vi "WT500 IEC 2015 Setup.vi"(0 "VISA Input":refnum<visa-resource-name>, 1 "Wiring (0: 1P2W, 1P2W, 1P2W)":T1=1 items=["1P2W, 1P2W, 1P2W", "1P3W, 1P2W", "3P3W, 1P2W", "1P2W, 1P3W", "1P2W, 3P3W", "3P4W", "3V3A"], 5 "V Range (8: 1000V)":u16(ring)=6 items=["AUTO", "15", "30", "60", "100", "150", "300", "600", "1000", "7.5", "15", "30", "50", "75", "150", "300", "500"], 7 "I Range (7: 40A)":u16(ring)=7 items=["AUTO", "500 mA", "1 A", "2 A", "5 A", "10 A", "20 A", "40 A", "S-AUTO", "50 mV", "100 mV", "200 mV", "500 mV", "1 V", "2 V", "5 V", "10 V", "250 mA", "500 mA", "1 A", "2.5 A", "5 A", "10 A", "20 A", "25 mV", "50 mV", "100 mV", "250 mV", "500 mV", "1 V", "2.5 V", "5 V"], 9 "Update Rate (3: 500ms)":u16(ring)=2 items=["-", "100ms", "200ms", "500ms", "1s", "2s", "5s"], 11 "Error In":errorcluster, 12 "Start/Stop (False: Stop)":bool=TRUE) -> (4 "VISA resource name out":refnum<visa-resource-name>, 6 "Standby Power Header":string[][](array[string]), 8 "WT500 Label Array":string[](array[string]), 10 "Uthd:Element 1":dbl, 15 "Error Out":errorcluster)   [LabVIEW 2019]
uses:
  Type Definitions/WT500 Wiring Control.ctl
  <vilib>/Utility/error.llb/whitespace.ctl
  <vilib>/Instr/_visa.llb/VISA Open Access Mode.ctl
  LLBs/ykwt500.llb/YKWT500 Read Numeric (Normal).vi
panel:
  in  "Pole":u16(ring)=1 items=["NONE", "Element 1", "Element 2", "Element 3", "Sigma"]
  in  "Measurement":u16(ring)=1 items=["None", "Urms", "Umn", "Udc", "Urmn", "Uac", "Irms", "Imn", "Idc", "Irmn", "Iac", "P", "S", "Q", "Lambda", "Phi", "Freq U", "Freq I", "U +peak", "U -peak", "I +peak", "I -peak", "Cf U", "Cf I", "Time", "Wp", "Wp+", "Wp-", "q", "q+", "q-", "WS", "WQ", "Eta 1", "Eta 2", "F1", "F2", "F3", "F4", "F5", "F6", "F7", "F8", "U(k)", "I(k)", "P(k)", "S(k)", "Q(k)", "Lambda(k)", "Phi(k)", "Phi U(k)", "Phi I(k)", "Uhdf(k)", "Ihdf(k)", "Phdf(k)", "Uthd", "Ithd", "Pthd", "Phi Ui-Uj", "Phi Ui-Uk", "Phi Ui-Ii", "Phi Ui-Ij", "Phi Ui-Ik", "Delta 1", "Delta 2", "Delta 3", "Delta 4"]
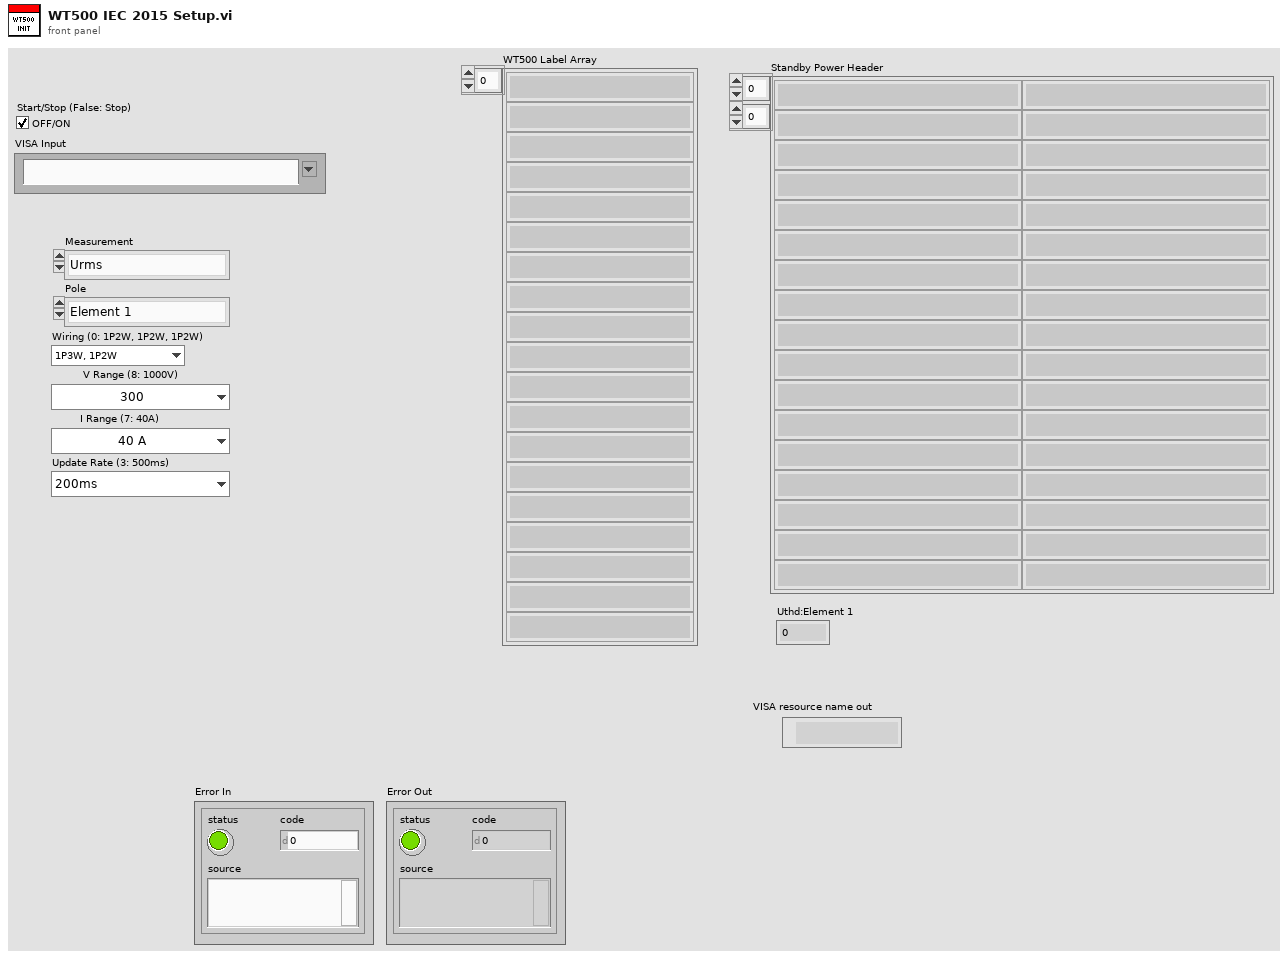
[diagram p1: front panel]
types:
  T1 = typedef "WT500 Wiring Control.ctl" = u16
  T2 = typedef "VISA Open Access Mode.ctl" = u32
  T3 = typedef "whitespace.ctl" = u16
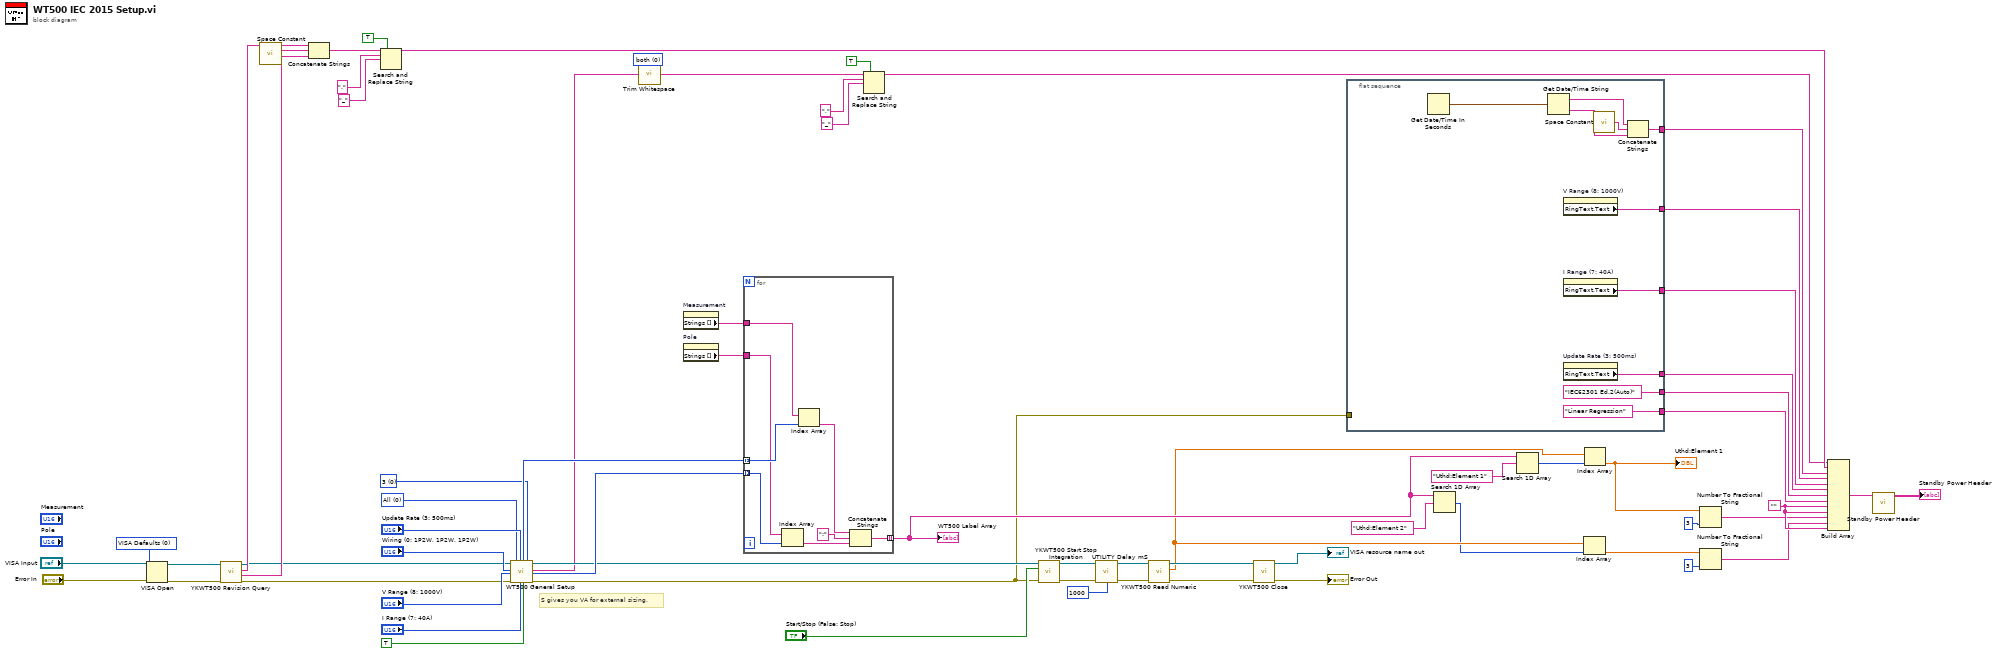
[diagram p0: block diagram]
diagram:
  w17 = T2 0 items=["VISA Defaults"=0, "Exclusive Lock"=1, "Load Configured Settings"=4] ("Access Mode")
  w18 = u16 0 items=["3", "6"] ("Crest Factor (0: 3)")
  w19 = u16 0 items=["All", "Element 1", "Element 2", "Element 3", "Sigma"] ("Element (0: All)")
  w25 = T3 0 items=["both", "start of string", "end of string"] ("location (both)")
  w45 = ""
  # "S gives you VA for external sizing."
  n1 = VISA Open(access mode=w17, error in (no error)="Error In", VISA resource name="VISA Input") -> (VISA resource name=w16:refnum<visa-resource-name>, error out=w15:errorcluster)  [unwired: 2 in]
  n2 = call "YKWT500 Revision Query.vi"("error in (no error)"=w15, "VISA resource name"=w16) -> ("error out"=w21:errorcluster, "Instrument Firmware Revision"=w52:string, "Instrument Driver Revision"=w53:string, "VISA resource name out"=w22:refnum<visa-resource-name>)  [unwired: 6 in]
  n3 = call <vilib>:"Space Constant.vi"() -> ("String"=w54:string)
  n4 = Concatenate Strings(w53, w54, w52) -> (w7:string)
  n5 = Search and Replace String(replace all?=TRUE ("replace all? (F)"), input string=w7, search string=",", replace string="_" ("replace string (\"\")")) -> (result string=w6:string)  [unwired: 4 in, 3 out]
  n6 = call "WT500 General Setup.vi"("VISA Refnum in"=w22, "Wiring (0: 1P2W, 1P2W, 1P2W)"="Wiring (0: 1P2W, 1P2W, 1P2W)", "V Range (8: 1000V)"="V Range (8: 1000V)", "error in (no error)"=w21, "Element (0: All)"=w19, "Update Rate (3: 500ms)"="Update Rate (3: 500ms)", "I Range (7: 40A)"="I Range (7: 40A)", "Reset Wh"=TRUE, "Crest Factor (0: 3)"=w18) -> ("Array of Measurements"=w63:u16[], "VISA Refnum out"=w58:refnum<visa-resource-name>, "Instrument ID"=w23:string, "Array Locations"=w64:u16[], "error out"=w26:errorcluster)  [unwired: 6 in]
  n7 = call <vilib>:"Trim Whitespace.vi"("string"=w23, "location (both)"=w25) -> ("trimmed string"=w2:string)
  n8 = property on="Measurement" class="Ring (strict)"() -> ("Strings []"=w60:string[])  [unwired: 2 in, 2 out]
  n9 = property on="Pole" class="Ring (strict)"() -> ("Strings []"=w59:string[])  [unwired: 2 in, 2 out]
  n10 = for {
    tunnel: w63 -> [w72] mode=indexing
    tunnel: w60 -> [w71]
    tunnel: w64 -> [w70] mode=indexing
    tunnel: w59 -> [w69]
    tunnel: [w65] -> w37 mode=indexing
    n11 = Index Array(array=w69, index=w70) -> (element=w66:string)
    n12 = Index Array(array=w71, index=w72) -> (element=w68:string)
    n13 = Concatenate Strings(w68, ":" ("string"), w66) -> (w65:string)
  }
  "WT500 Label Array" <- w37
  n14 = Search and Replace String(replace all?=TRUE ("replace all? (F)"), input string=w2, search string=",", replace string="_" ("replace string (\"\")")) -> (result string=w1:string)  [unwired: 4 in, 3 out]
  n15 = call "YKWT500 Start Stop Integration.vi"("error in (no error)"=w26, "Start/Stop (False: Stop)"="Start/Stop (False: Stop)", "VISA resource name"=w58) -> ("error out"=w29:errorcluster, "VISA resource name out"=w44:refnum<visa-resource-name>)  [unwired: 7 in]
  n16 = call "UTILITY Delay mS.vi"("Error In"=w29, "milliseconds to wait"=u32 1000) -> ("Error Out"=w28:errorcluster)  [unwired: 13 in]
  n17 = call-poly "YKWT500 Read Numeric.vi"("error in (no error)"=w28, "VISA resource name"=w44) -> ("error out"=w43:errorcluster, "Measurement Value"=w36:dbl[], "VISA resource name out"=w42:refnum<visa-resource-name>)  [unwired: 7 in]
  "VISA resource name out" <- w42
  n18 = call "YKWT500 Close.vi"("error in (no error)"=w43, "VISA resource name"=w42) -> ("error out"=→"Error Out":errorcluster)  [unwired: 9 in]
  n19 = flat-sequence {
    tunnel: [w78] -> w51
    tunnel: [w75] -> w50
    tunnel: [w74] -> w49
    tunnel: [w73] -> w48
    tunnel: ["IEC62301 Ed.2(Auto)" ("element")] -> w47
    tunnel: ["Linear Regression" ("element")] -> w46
    tunnel: w26 -> [_]
    frame #0 {
      n20 = Get Date/Time In Seconds() -> (seconds since 1Jan1904=w79:timestamp)
      n21 = Get Date/Time String(seconds (now)=w79) -> (date string=w81:string, time string=w82:string)  [unwired: 2 in]
      n22 = property on="V Range (8: 1000V)" class="Ring (strict)"() -> ("RingText.Text"=w75:string)  [unwired: 2 in, 2 out]
      n23 = property on="I Range (7: 40A)" class="Ring (strict)"() -> ("RingText.Text"=w74:string)  [unwired: 2 in, 2 out]
      n24 = property on="Update Rate (3: 500ms)" class="Ring (strict)"() -> ("RingText.Text"=w73:string)  [unwired: 2 in, 2 out]
      n25 = call <vilib>:"Space Constant.vi"() -> ("String"=w80:string)
      n26 = Concatenate Strings(w81, w80, w82) -> (w78:string)
    }
  }
  n27 = Search 1D Array(1D array=w37, element="Uthd:Element 2") -> (index of element=w34:i32)  [unwired: 1 in]
  n28 = Search 1D Array(1D array=w37, element="Uthd:Element 1") -> (index of element=w35:i32)  [unwired: 1 in]
  n29 = Index Array(array=w36, index=w34) -> (element=w32:dbl)
  n30 = Index Array(array=w36, index=w35) -> (element=w33:dbl)
  "Uthd:Element 1" <- w33
  n31 = Number To Fractional String(number=w33, precision (6)=i16 3) -> (F-format string=w31:string)  [unwired: 2 in]
  n32 = Number To Fractional String(number=w32, precision (6)=i16 3) -> (F-format string=w30:string)  [unwired: 2 in]
  n33 = Build Array(w1, w6, w51, w50, w49, w48, w47, w46, w45, w45, w31, w30, w45) -> (w12:string[])
  n34 = call "Standby Power Header.vi"("Array"=w12) -> ("Header File"=→"Standby Power Header":string[][])  [unwired: 9 in, 1 out]
